vi "NI 5772 (AC) - Digitizer_vDirectDataSend (FPGA) Averaging (Working).vi"() -> ()   [LabVIEW 2020]
doc: "Example Description:\nThis example demonstrates how to enable Time Interleaved Sampling with the NI 5772 adapter module to achieve a sampling rate of 1.6GS/s. This example continuously acquires records of analog input data from the NI 5772 adapter module. It allows you to select an AI channel, trigger type, and record size. This VI must be compiled before it is run. \n\nRunning the VI:\nThis VI must be run from the NI 5772 - Getting Started (Host).vi. Refer to the host VI documentation for steps regarding running and configuring the FPGA VI. \n\nExecution Steps:\nRefer to the Block Diagram of this VI for execution comments."
uses:
  Controls/AI Trigger Type.ctl
  Controls/Aquire State.ctl
  <vilib>/Platform/TimedLoop/XDataNode/timing_clust.ctl
  <vilib>/Platform/TimedLoop/XDataNode/nitl_modes.ctl
  <vilib>/Platform/TimedLoop/XDataNode/wakeup.ctl
  Controls/DigitizerState.ctl
  <vilib>/rvi/Emulation/niFpgaGetClockAttributes.vi
  <vilib>/rvi/Emulation/niFpgaSctlEmulationGetInTimedLoop.vi
  <vilib>/rvi/Emulation/niFpgaEmulationReportErrorSimple.vi
  <vilib>/rvi/eio/common/nirviEmuTemplateMethod_errors.vi
  <vilib>/rvi/Emulation/niFpgaCriticalErrorInLSC.vi
  <vilib>/rvi/Emulation/niFpgaProcessEmulError.vi
  <vilib>/rvi/Emulation/niFpgaEmulationIsFPGAContextNoSignature.vi
  <vilib>/rvi/errors/niFpgaSetErrorForExecOnDevCompSimple.vi
  <vilib>/rvi/eio/common/nirviEmuReportErrorAndStop.vi
  <vilib>/rvi/DataTransferAndStorage/Container/Common/niFpgaContainerGetUniqueNameForEmu.vi
  <vilib>/rvi/FIFO/Fifo_Resource/nirvififoEmulationSetSize.vi
  <vilib>/rvi/FIFO/Fifo_Resource/nirviFifoEmulationQueueMgr.vi
  <instcachedir>/0/nirviFifoEmulationQueueMgr_E5CAEC123FF24DC58D834DCA3CDAA9B5.lvgen/nirviFifoEmulationQueueMgr_E5CAEC123FF24DC58D834DCA3CDAA9B5_004.vi
  <vilib>/Utility/error.llb/Clear Errors.vi
  <vilib>/rvi/FIFO/Fifo_Resource/nirvififoEmulationCreateLock.vi
  <vilib>/rvi/FIFO/Fifo_Resource/nirvififoEmulationObtainLock.vi
  <vilib>/rvi/FIFO/Fifo_Resource/nirvififoEmulationReleaseLock.vi
  <vilib>/rvi/occurrence/nirviWaitOnOccurrenceBase.vi
  <vilib>/rvi/errors/nirviReportUnexpectedCaseInternalError.vi
  <vilib>/rvi/errors/nirviReportUnexpectedCaseInternalError (U32).vi
  <instcachedir>/0/nirviFifoEmulationQueueMgr_E5CAEC123FF24DC58D834DCA3CDAA9B5.lvgen/nirviFifoEmulationQueueMgr_E5CAEC123FF24DC58D834DCA3CDAA9B5_000.vi
  <instcachedir>/0/nirviFifoEmulationQueueMgr_E5CAEC123FF24DC58D834DCA3CDAA9B5.lvgen/nirviFifoEmulationQueueMgr_E5CAEC123FF24DC58D834DCA3CDAA9B5_003.vi
  <vilib>/rvi/FIFO/Fifo_Resource/nirvififoEmulationDetermineInputValidOut.vi
  <vilib>/rvi/Memory/Memory_Emulation/nirvimemoryFastEmulation.vi
  <vilib>/rvi/Memory/Memory_Emulation/nirvimemoryEmulation.vi
  <vilib>/rvi/interface/RandomDataEmulation/niFpgaRandomDataHandleErrors.vi
  <instrlib>/_niInstr/Basic Elements/v1/FPGA/Private/Count Up U64.vi
  <vilib>/eio/EIONode/EIONode.xnode
  <vilib>/rvi/DataTransferAndStorage/Container/XNode/niFpgaContainer.xnode
  <vilib>/rvi/FIFO/Fifo_Resource/nirvififoEmulationRead.vi
  <vilib>/Platform/TimedLoop/XDataNode/XDataNode.xnode
  <vilib>/rvi/FIFO/Fifo_Resource/nirvififoEmulationWrite.vi
  <vilib>/rvi/interface/RandomDataEmulation/nirviRandomDataFpgaReadWriteTemplate.vi
  <vilib>/Platform/TimedLoop/XDataNode/XDNodeRunTimeDep.lvlib
  <instrlib>/_niInstr/Basic Elements/v1/FPGA/niInstr Basic Elements v1 FPGA.lvlib
panel:
  out "Read Size (Host)":u16=512 caption="Samples Per Trigger" min=1 step=1
  out "Trig Count":u64
  in  "Clear Count":bool
  in  "TrigIn Simulate":bool
  in  "vi/nGenTrig":bool
  in  "Arm Trigger":bool
  out "F to H FIFO Overflow?":bool caption="FIFO Overflow?"
  out "DataAlignmentFIFO":bool
  out "Aq to Trans FIFO Overflow?":bool caption="FIFO Overflow?"
  in  "Requested Samples Per Pixel":u16=512 caption="Samples Per Trigger" min=1 step=1
  in  "AvgCount_powerOf2":i16=1
  in  "Delay (us)":sgl
  in  "WaveSampleCount":sgl=256.0 format="%#_13g"
  in  "Wave Sampling Rate":sgl=200000000.0 format="%#_6p"
  in  "Trigger Level":i16
  in  "Trigger Type":T1
  out "AvgCount":u16=1
  out "Delay after Trig [cycles]":u16
  out "1/8th Samples Per Trigger":u16=512 caption="Samples Per Trigger" min=1 step=1
  out "WaitForWave\nCompletion [cycles]":u16
  in  "User Command Commit":bool
  in  "User Command":u8
  out "User Command Idle":bool
  out "User Command Status":u8
  in  "User Data 0":u16
  in  "User Data 1":u8
  out "PLL Locked":bool
  out "User Error":bool
  out "Configured?":bool
  # "Trigger Settings"
  # "FIFO Status"
  # "Analog Input"
  # "Clock Configuration"
  # "Resource Configuration"
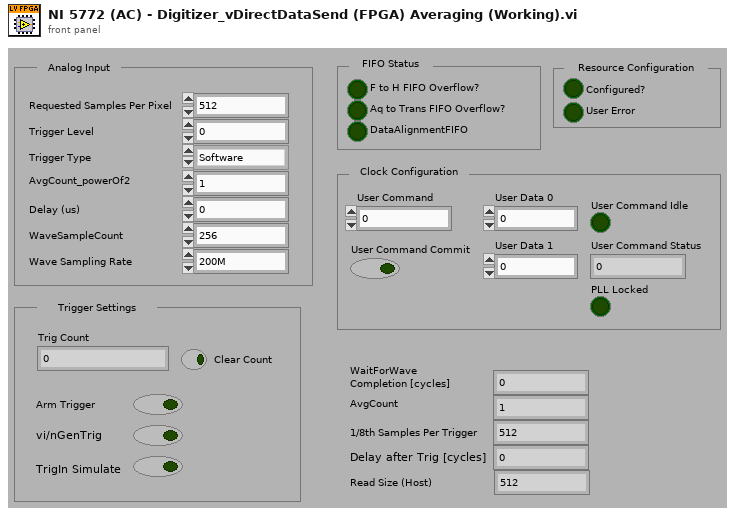
[diagram p1: front panel]
types:
  T1 = typedef "AI Trigger Type.ctl" = enum8{"Software", "Data Edge"}
  T2 = typedef "DigitizerState.ctl" = enum16{"Init", "Build/Clear Accumulator", "GetData", "SetData", "AverageCountCheck", "SendtoHost"}
  T3 = typedef "Aquire State.ctl" = enum8{"Idle", "Wait for Trigger", "AlignWave", "Hold Aquire", "Acquire", "WaitForWaveCompletion", "CheckAvg"}
  T4 = typedef "XDNodeRunTimeDep.lvlib/timing_clust.ctl" = cluster{"Expected End [f-1]":u64, "Actual End [f-1]":u64, "Finished Late? [f-1]":bool, "Expected End [i-1]":u64, "Actual End [i-1]":u64, "Finished Late? [i-1]":bool, "Expected Start [i]":u64, "Actual Start [i]":u64, "Expected Start [f]":u64, "Actual Start [f]":u64, "Source Name":string, "Structure Name":string, "Period":i64, "Deadline":i64, "Offset":i64, "Start":i64, "Priority":i32, "Timeout":i32, "Mode":T5, "Wakeup Reason":T6, "Error":errorcluster, "Source Type":string, "Secondary Source Type":string, "Global End Time":u64, "Global Start Time":u64, "Frame Duration":u64, "Iteration Duration":u64, "Assigned CPU":i32, "I/O Scan Engine Mode":u32}
  T5 = typedef "XDNodeRunTimeDep.lvlib/nitl_modes.ctl" = enum32{"No Change", "Process missed periods, maintain original phase", "Discard missed periods, maintain original phase", "Process missed periods, ignore original phase", "Discard missed periods, ignore original phase"}
  T6 = typedef "XDNodeRunTimeDep.lvlib/wakeup.ctl" = enum32{"Normal", "Aborted", "Asynchronous wakeup", "Timing source error", "Timed loop error", "Timeout"}
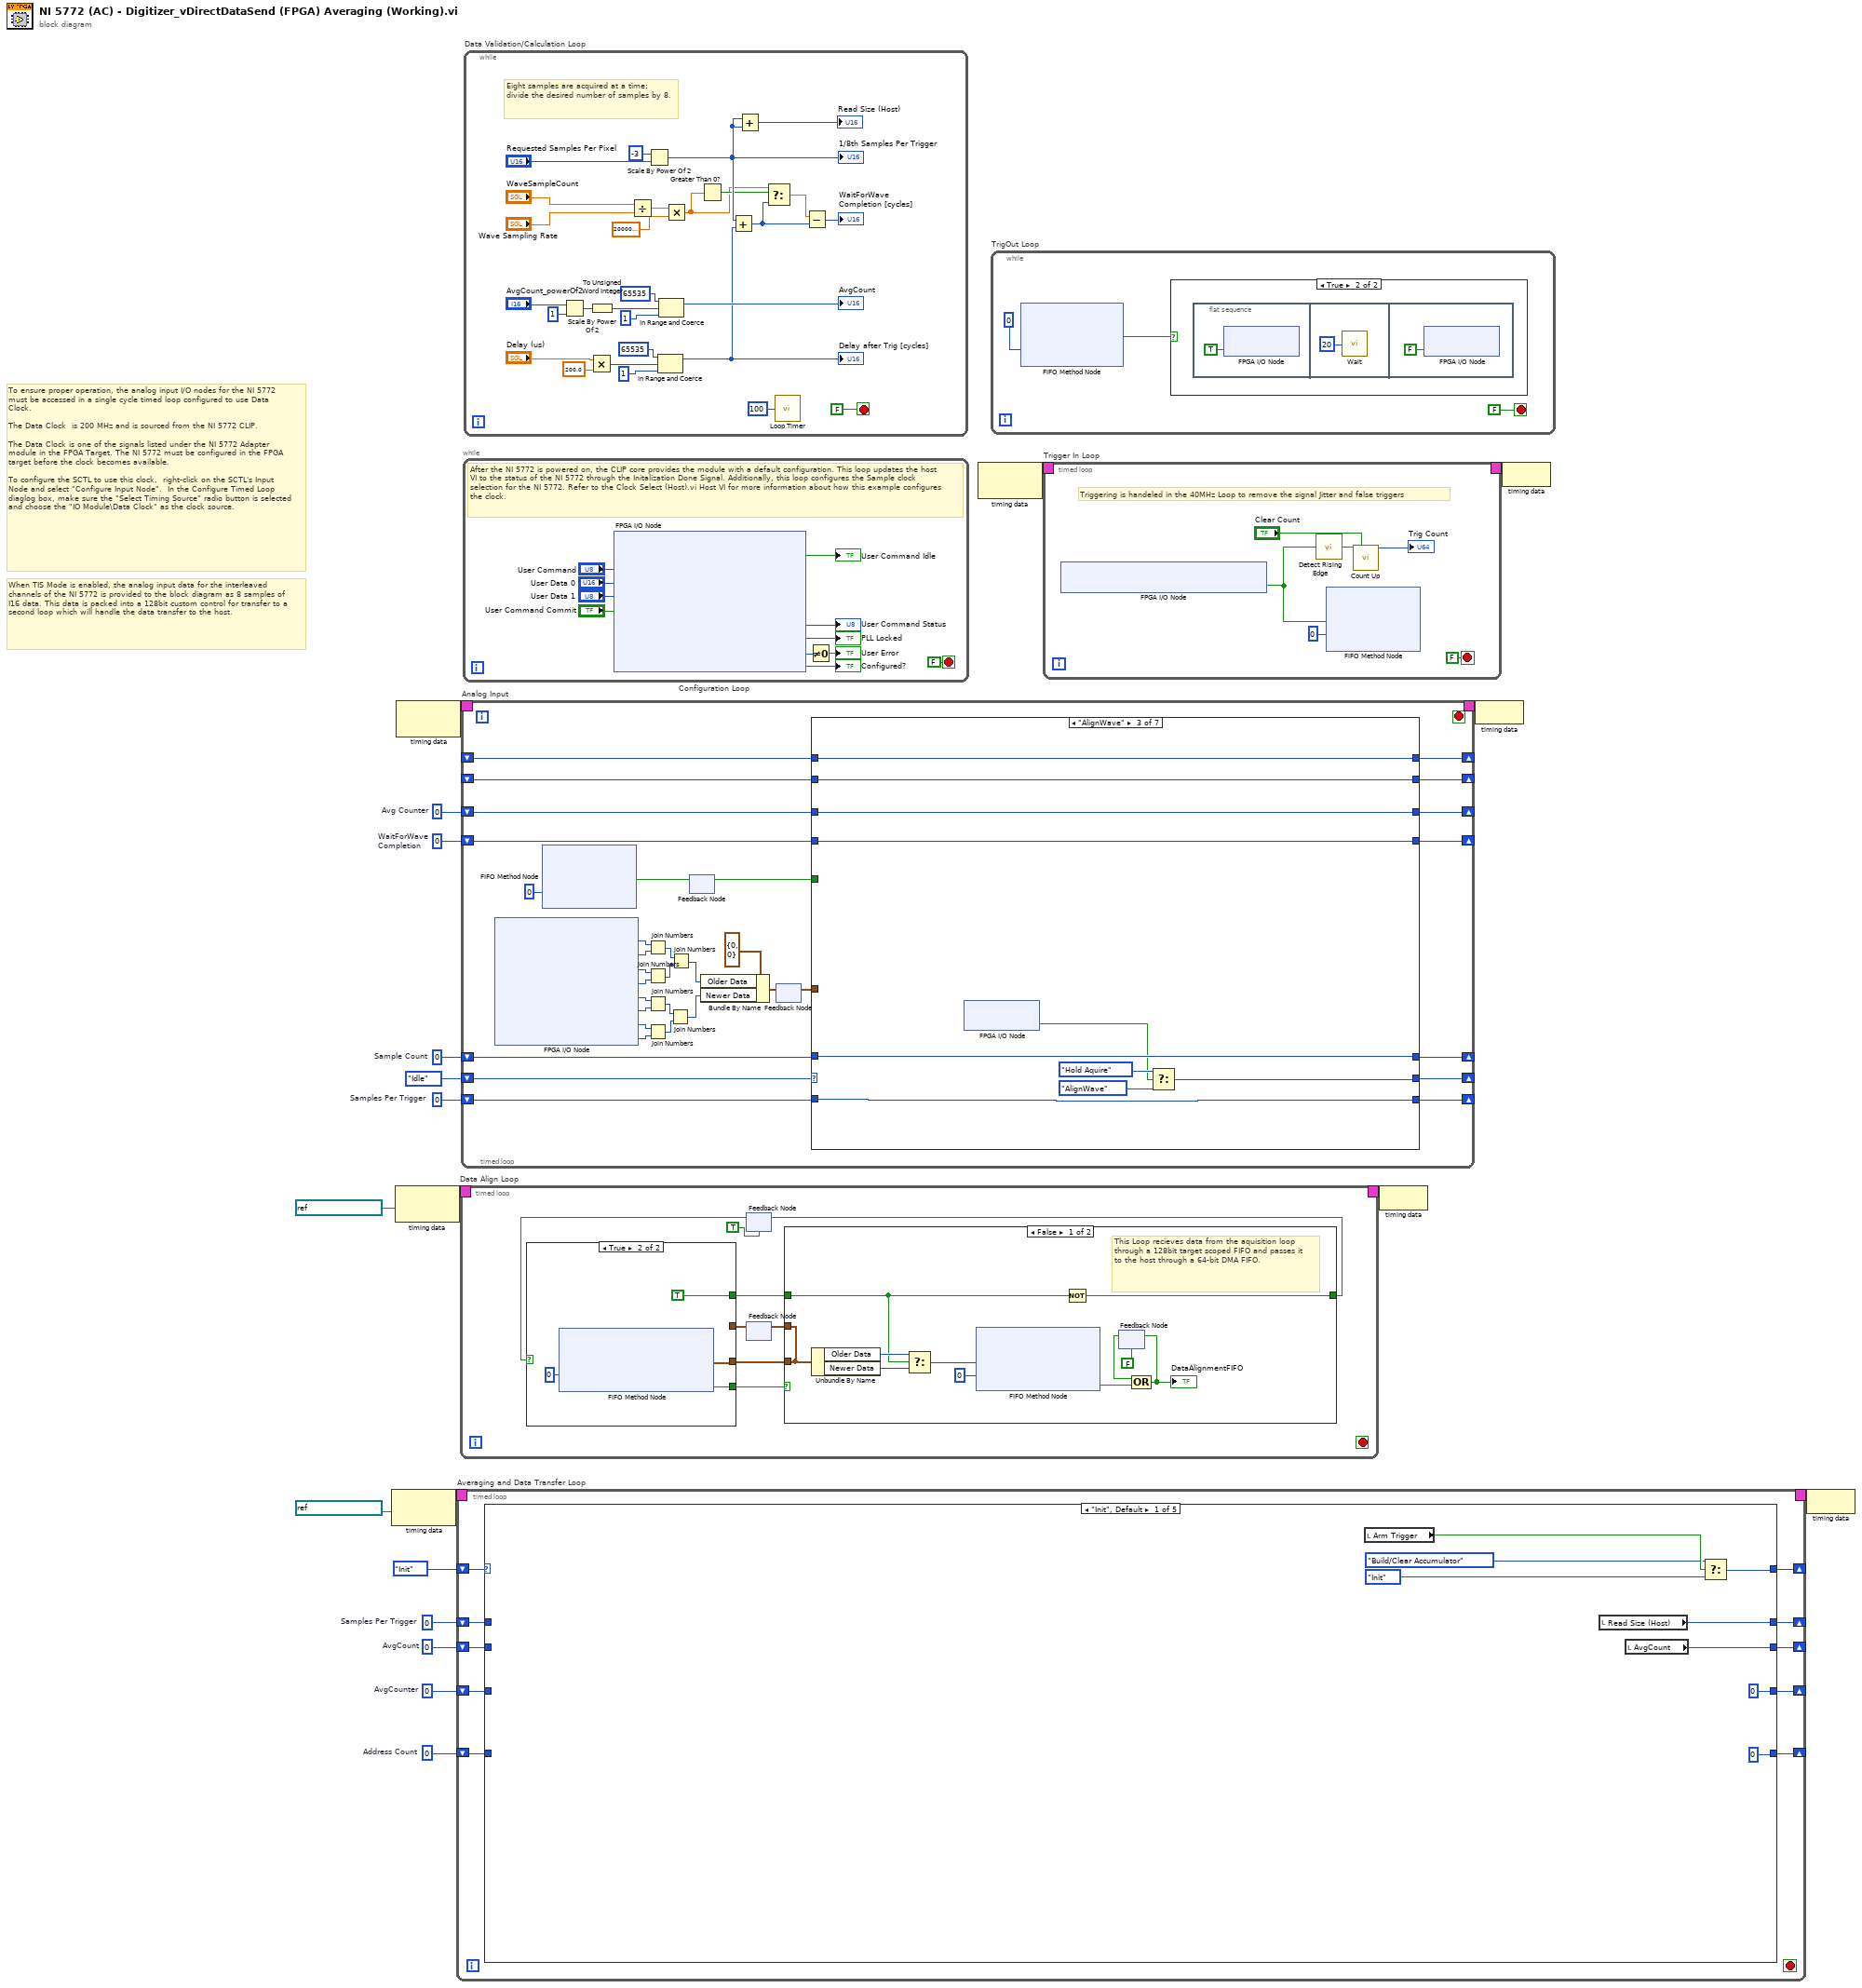
[diagram p0: block diagram]
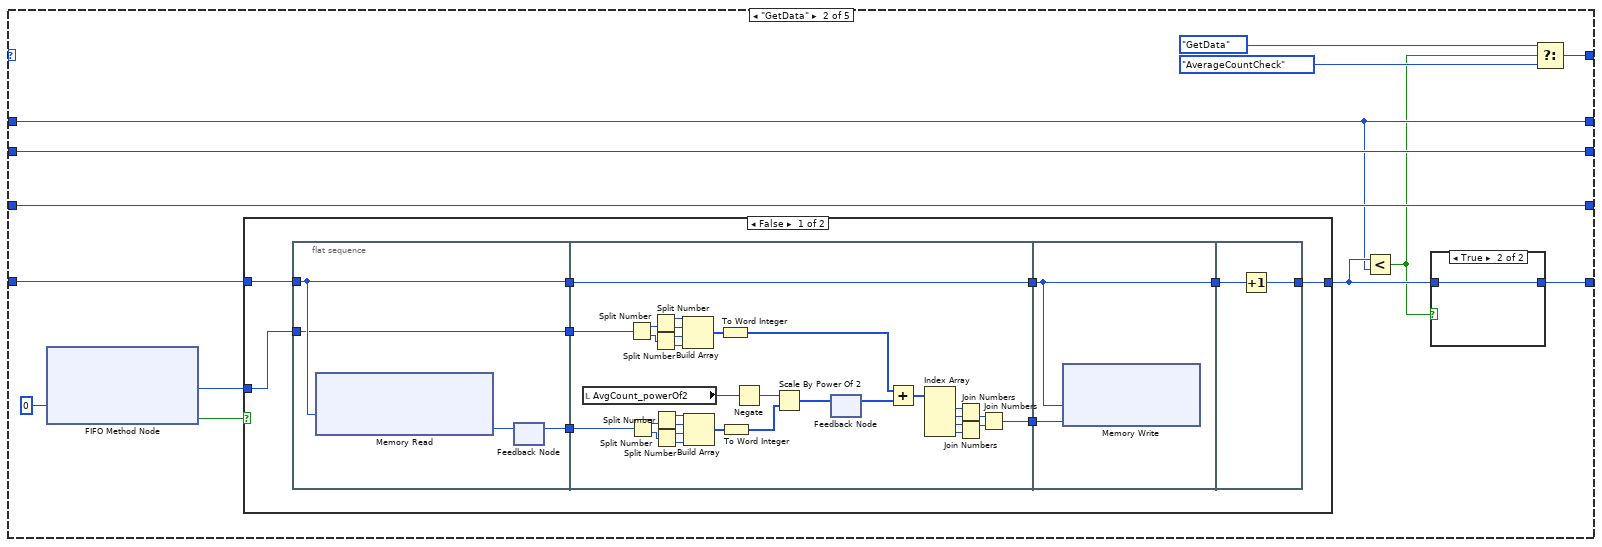
[diagram p2: hidden frame]
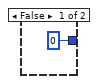
[diagram p3: hidden frame]
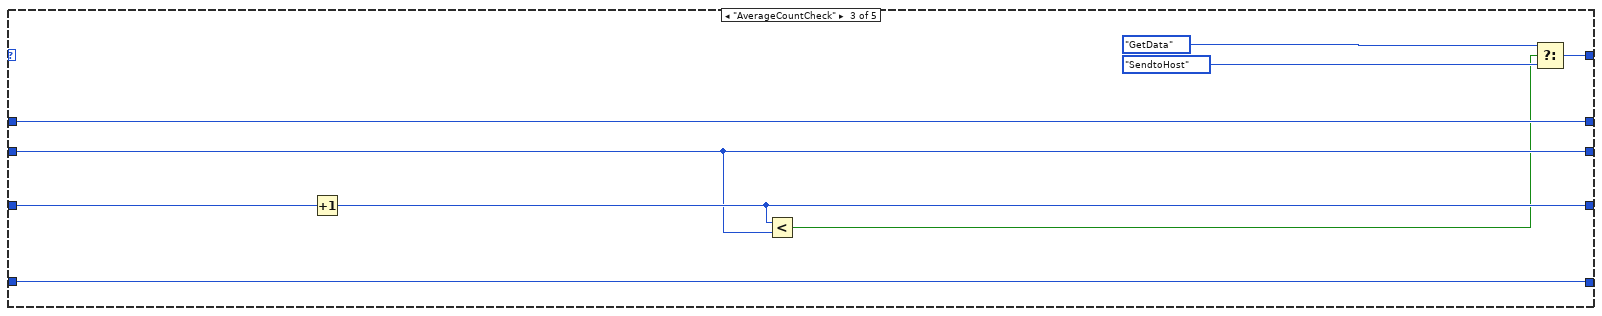
[diagram p5: hidden frame]
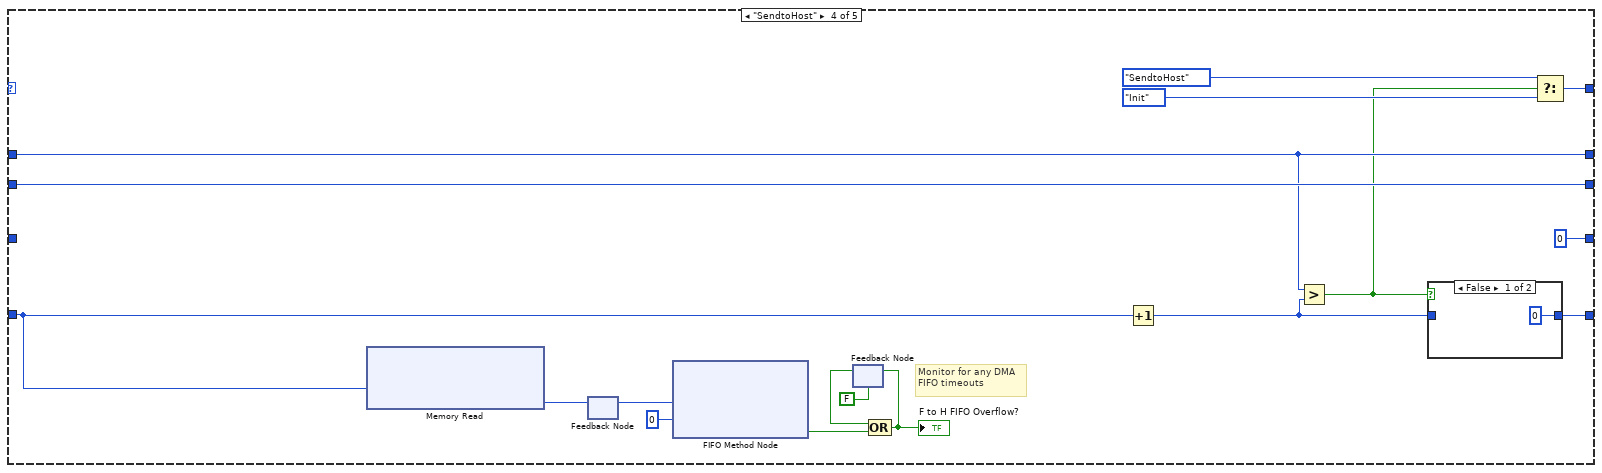
[diagram p6: hidden frame]
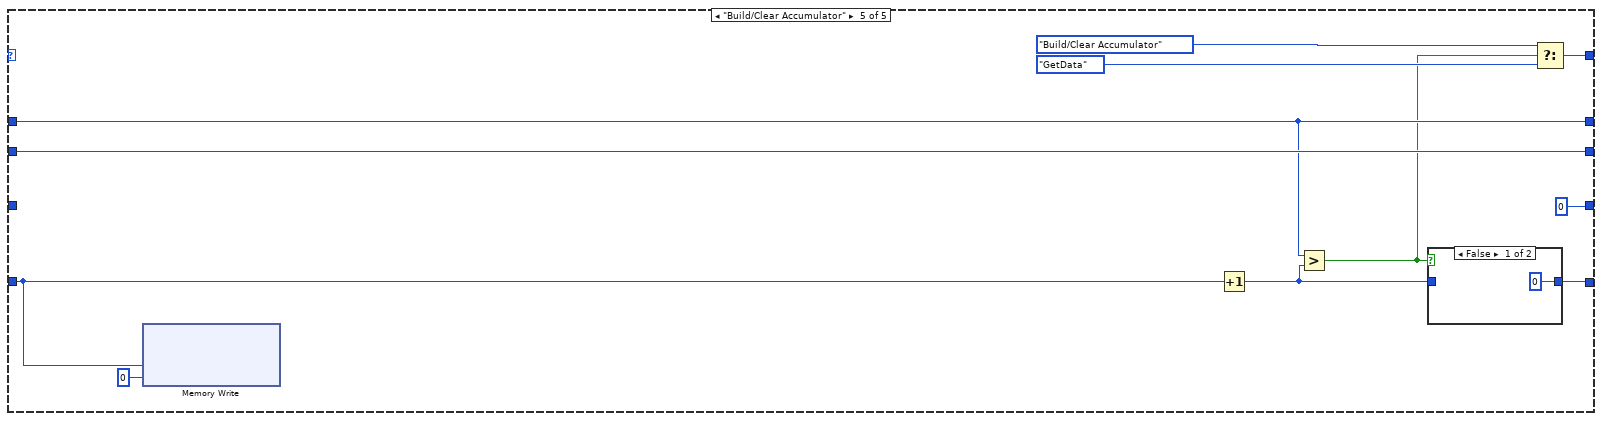
[diagram p8: hidden frame]
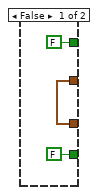
[diagram p10: hidden frame]
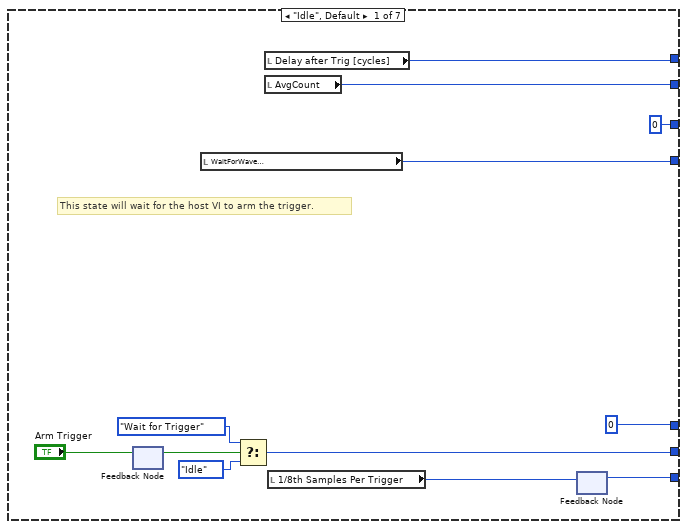
[diagram p13: hidden frame]
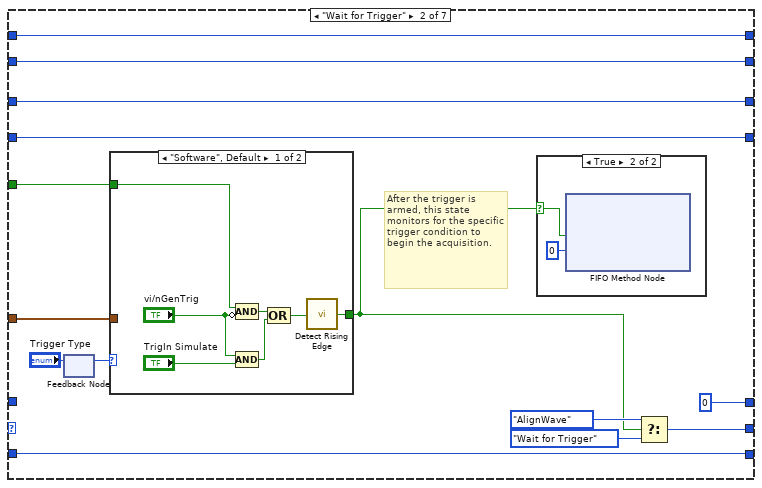
[diagram p14: hidden frame]
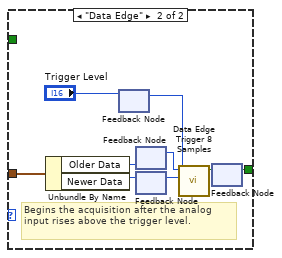
[diagram p16: hidden frame]
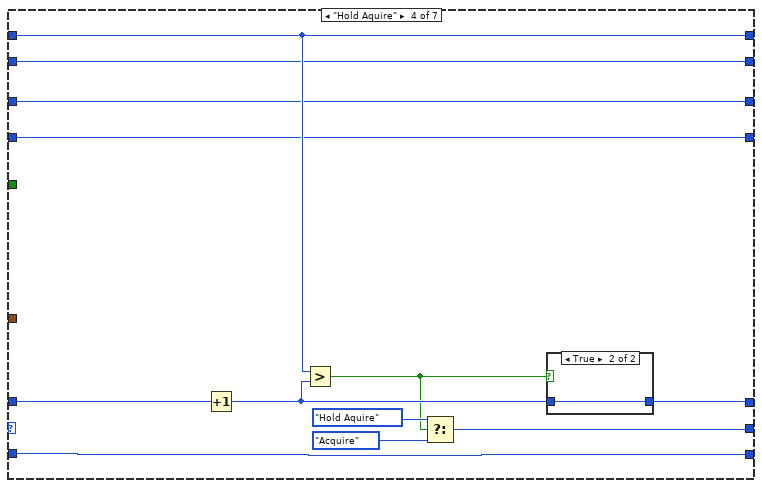
[diagram p17: hidden frame]
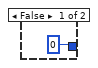
[diagram p18: hidden frame]
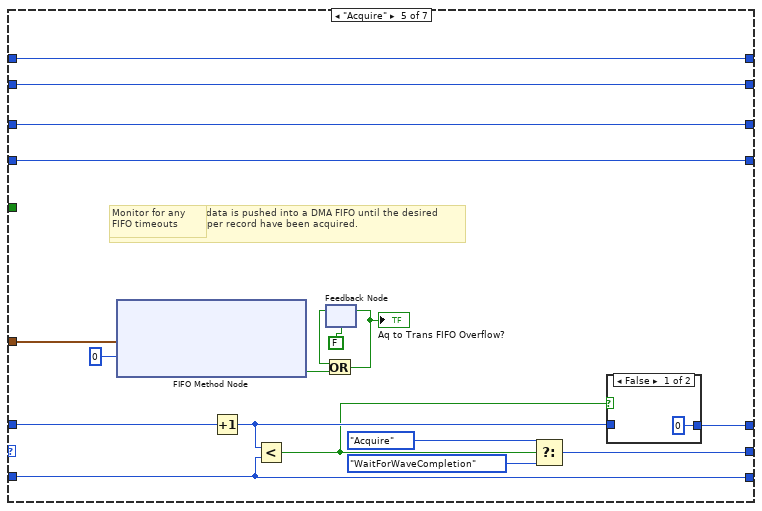
[diagram p19: hidden frame]
diagram:
  w6 = u16 0  # AvgCounter
  w5 = u32 0  # Address Count
  w4 = u16 0  # AvgCount
  w3 = u16 0  # Samples Per Trigger
  w12 = u16 0  # WaitForWave Completion
  w13 = u16 0  # Avg Counter
  w14 = u16 0  # Samples Per Trigger
  w15 = u16 0  # Sample Count
  # "When TIS Mode is enabled, the analog input data for the interleaved channels of the NI 5772 is provided to the block diagram as 8 samples of I16 data. This data is packed into a 128bit custom control for transfer to a second loop which will handle the data transfer to the host."
  # "To ensure proper operation, the analog input I/O nodes for the NI 5772 must be accessed in a single cycle timed loop configured to use Data Clock. \n\nThe Data Clock  is 200 MHz and is sourced from the NI 5772 CLIP.\n\nThe Data Clock is one of the signals listed under the NI 5772 Adapter module in the FPGA Target. The NI 5772 must be configured in the FPGA target before the clock becomes available. \n\nTo configure the SCTL to use this clock,  right-click on the SCTL's Input Node and select \"Configure Input Node\".  In the Configure Timed Loop diaglog box, make sure the \"Select Timing Source\" radio button is selected and choose the \"IO Module\\Data Clock\" as the clock source."
  n1 = node-c288(refnum<k21> "100 MHz Clock" ("Source Name")) -> (w8:T4)
  n2 = node-c288(refnum<k21> "100 MHz Clock" ("Source Name")) -> (w11:T4)
  n3 = node-c288() -> (w20:T4)  [unwired: 1 in]
  n4 = timed-loop "Averaging and Data Transfer Loop" {
    timing: w8 -> [_]
    timing-out: [_] -> w7
    shift-right: [w29] -> _
    shift-left: DigitizerState."Init" -> [w30]
    shift-right: [w28] -> _
    shift-left: w3 -> [w26]
    shift-right: [w27] -> _
    shift-left: w4 -> [w25]
    shift-right: [w23] -> _
    shift-left: w5 -> [w24]
    shift-right: [w21] -> _
    shift-left: w6 -> [w22]
    stop <- _ stop-if-true
    n5 = case shown="\"Init\", Default" w30 {
      tunnel: [w34 w49 w109 w125 w138] -> w29
      tunnel: [w32 w41 w107 w123 w136] -> w28
      tunnel: [w35 w48 w104 w128 w141] -> w27
      tunnel: w26 -> [_ w41 w107 w123 w136]
      tunnel: w25 -> [_ w48 w104 w128 w141]
      tunnel: w24 -> [_ w44 w108 w113 w132]
      tunnel: [u32 0 w43 w108 w124 w137] -> w23
      tunnel: [u16 0 w46 w105 u16 0 ("AvgCounter") u16 0 ("AvgCounter")] -> w21
      tunnel: w22 -> [_ w46 w106 _ _]
      frame "Init", Default {
        n6 = local read "Arm Trigger"() -> (w38:bool)
        n7 = local read "Read Size (Host)"() -> (w32:u16)
        n8 = local read "AvgCount"() -> (w35:u16)
        n9 = Select(t=DigitizerState."Build/Clear Accumulator", s=w38, f=DigitizerState."Init") -> (s? t:f=w34:T2)
      }
      frame "GetData" {
        n10 = xnode ("FIFO Method Node")("Timeout"=0) -> ("Element"=w45:u64, "Timed Out?"=w40:bool)  [unwired: 1 in, 1 out]
        n11 = case shown="False" w40 {
          tunnel: w45 -> [w59 _]
          tunnel: w44 -> [w61 w102]
          tunnel: [w58 w102] -> w42
          frame False {
            n12 = flat-sequence {
              tunnel: [w65] -> w62
              tunnel: w61 -> [w64]
              tunnel: w59 -> [w63]
              tunnel: [w64] -> w57
              tunnel: [w63] -> w55
              tunnel: w62 -> [w68]
              tunnel: [w87] -> w60
              tunnel: w57 -> [w86]
              tunnel: [w86] -> w56
              tunnel: w55 -> [w77]
              tunnel: w60 -> [w99]
              tunnel: w56 -> [w98]
              tunnel: [w98] -> w54
              tunnel: [w100] -> w58
              tunnel: w54 -> [w101]
              frame #0 {
                n13 = xnode ("Memory Read")("Address"=w64) -> ("Data"=w66:u64)  [unwired: 1 in, 1 out]
                n14 = feedback #1() -> (w65:u64)  [unwired: 1 in]
                n15 = feedback-in #1(w66) -> ()
              }
              frame #1 {
                n16 = local read "AvgCount_powerOf2"() -> (w96:i16)
                n17 = Split Number(x=w77) -> (hi(x)=w84:u32, lo(x)=w83:u32)
                n18 = Split Number(x=w68) -> (hi(x)=w69:u32, lo(x)=w70:u32)
                n19 = Split Number(x=w84) -> (hi(x)=w82:u16, lo(x)=w81:u16)
                n20 = Split Number(x=w83) -> (hi(x)=w80:u16, lo(x)=w79:u16)
                n21 = Split Number(x=w69) -> (hi(x)=w71:u16, lo(x)=w72:u16)
                n22 = Split Number(x=w70) -> (hi(x)=w73:u16, lo(x)=w74:u16)
                n23 = Build Array(w82, w81, w80, w79) -> (w78:u16[])
                n24 = Build Array(w71, w72, w73, w74) -> (w75:u16[])
                n25 = To Word Integer(number=w78) -> (16bit integer=w76:i16[])
                n26 = To Word Integer(number=w75) -> (16bit integer=w67:i16[])
                n27 = Negate(x=w96) -> (-x=w97:i16)
                n28 = Scale By Power Of 2(n=w97, x=w67) -> (x*2^n=w95:i16[])
                n29 = feedback-in #2(w95) -> ()
                n30 = feedback #2() -> (w85:i16[])  [unwired: 1 in]
                n31 = Add(x=w76, y=w85) -> (x+y=w88:i16[])
                n32 = Index Array(array=w88) -> (element #1=w91:i16, element #2=w92:i16, element #3=w93:i16, element #4=w94:i16)  [unwired: 4 in]
                n33 = Join Numbers(hi=w91, lo=w92) -> ((hi.lo)=w89:u32)
                n34 = Join Numbers(hi=w93, lo=w94) -> ((hi.lo)=w90:u32)
                n35 = Join Numbers(hi=w89, lo=w90) -> ((hi.lo)=w87:u64)
              }
              frame #2 {
                n36 = xnode ("Memory Write")("Address"=w98, "Data"=w99) -> ()  [unwired: 1 in, 1 out]
              }
              frame #3 {
                n37 = Increment(x=w101) -> (x+1=w100:u32)
              }
            }
          }
          frame True {
          }
        }
        n38 = Less?(x=w42, y=w41) -> (x < y?=w39:bool)
        n39 = case shown="True" w39 {
          tunnel: w42 -> [_ w53]
          tunnel: [u32 0 w53] -> w43
          frame False {
          }
          frame True {
          }
        }
        n40 = Select(t=DigitizerState."GetData", s=w39, f=DigitizerState."AverageCountCheck") -> (s? t:f=w49:T2)
      }
      frame "AverageCountCheck" {
        n41 = Increment(x=w106) -> (x+1=w105:u16)
        n42 = Less?(x=w105, y=w104) -> (x < y?=w103:bool)
        n43 = Select(t=DigitizerState."GetData", s=w103, f=DigitizerState."SendtoHost") -> (s? t:f=w109:T2)
      }
      frame "SendtoHost" {
        # "Monitor for any DMA FIFO timeouts"
        n44 = xnode ("Memory Read")("Address"=w113) -> ("Data"=w114:u64)  [unwired: 1 in, 1 out]
        n45 = feedback #3() -> (w112:u64)  [unwired: 1 in]
        n46 = feedback-in #3(w114) -> ()
        n47 = xnode ("FIFO Method Node")("Element"=w112, "Timeout"=0) -> ("Timed Out?"=w119:bool)  [unwired: 1 in, 1 out]
        n48 = feedback #4(FALSE) -> (w118:bool)
        n49 = Compound Arithmetic op=OR(w118, w119) -> (w120:bool)
        "F to H FIFO Overflow?" <- w120
        n50 = feedback-in #4(w120) -> ()
        n51 = Increment(x=w113) -> (x+1=w122:u32)
        n52 = Greater?(x=w123, y=w122) -> (0:w121:bool)
        n53 = case shown="False" w121 {
          tunnel: w122 -> [_ w130]
          tunnel: [u32 0 w130] -> w124
          frame False {
          }
          frame True {
          }
        }
        n54 = Select(t=DigitizerState."SendtoHost", s=w121, f=DigitizerState."Init") -> (s? t:f=w125:T2)
      }
      frame "Build/Clear Accumulator" {
        n55 = xnode ("Memory Write")("Address"=w132, "Data"=u64 0) -> ()  [unwired: 1 in, 1 out]
        n56 = Increment(x=w132) -> (x+1=w135:u32)
        n57 = Greater?(x=w136, y=w135) -> (0:w134:bool)
        n58 = case shown="False" w134 {
          tunnel: w135 -> [_ w143]
          tunnel: [u32 0 w143] -> w137
          frame False {
          }
          frame True {
          }
        }
        n59 = Select(t=DigitizerState."Build/Clear Accumulator", s=w134, f=DigitizerState."GetData") -> (s? t:f=w138:T2)
      }
    }
  }
  n60 = timed-loop "Data Align Loop" {
    timing: w11 -> [_]
    timing-out: [_] -> w10
    stop <- _ stop-if-true
    n61 = feedback #5(TRUE ("Timed Out?")) -> (w148:bool)
    n62 = feedback #6() -> (w149:cluster{"Older Data":u64, "Newer Data":u64})  [unwired: 1 in]
    n63 = case shown="True" w148 {
      tunnel: [w154 w157] -> w151
      tunnel: [FALSE ("Timed Out?") w158] -> w153
      tunnel: [FALSE ("Timed Out?") TRUE ("Timed Out?")] -> w152
      tunnel: w149 -> [w154 _]
      frame False {
      }
      frame True {
        n64 = xnode ("FIFO Method Node")("Timeout"=0) -> ("Element"=w157:cluster{"Older Data":u64, "Newer Data":u64}, "Timed Out?"=w158:bool)  [unwired: 1 in, 1 out]
      }
    }
    n65 = case shown="False" w153 {
      tunnel: [w169 w173] -> w147
      tunnel: w152 -> [w170 w173]
      tunnel: w151 -> [w168 w172]
      tunnel: [w168 w172] -> w150
      frame False {
        # "This Loop recieves data from the aquisition loop through a 128bit target scoped FIFO and passes it to the host through a 64-bit DMA FIFO."
        n66 = Unbundle By Name(w168) -> ("Older Data"=w171:u64, "Newer Data"=w167:u64)
        n67 = Select(t=w171, s=w170, f=w167) -> (s? t:f=w161:u64)
        n68 = xnode ("FIFO Method Node")("Element"=w161, "Timeout"=0) -> ("Timed Out?"=w163:bool)  [unwired: 1 in, 1 out]
        n69 = Not(x=w170) -> (.not. x?=w169:bool)
        n70 = feedback #7(FALSE) -> (w164:bool)
        n71 = Compound Arithmetic op=OR(w164, w163) -> (w162:bool)
        "DataAlignmentFIFO" <- w162
        n72 = feedback-in #7(w162) -> ()
      }
      frame True {
      }
    }
    n73 = feedback-in #5(w147) -> ()
    n74 = feedback-in #6(w150) -> ()
  }
  n75 = timed-loop "Analog Input" {
    timing: w20 -> [_]
    timing-out: [_] -> w19
    shift-right: [w208] -> _
    shift-left: Aquire_State."Idle" ("Acquire State") -> [w198]
    shift-right: [w209] -> _
    shift-left: w15 -> [w199]
    shift-right: [w207] -> _
    shift-left: w14 -> [w197]
    shift-right: [w184] -> _
    shift-left: _ -> [w183]
    shift-right: [w182] -> _
    shift-left: _ -> [w181]
    shift-right: [w179] -> _
    shift-left: w13 -> [w180]
    shift-right: [w177] -> _
    shift-left: w12 -> [w176]
    stop <- _ stop-if-true
    n76 = xnode "FPGA I/O Node"() -> ("IO Module\\AI 1 Data N-3"=w190:i16, "IO Module\\AI 0 Data N-3"=w189:i16, "IO Module\\AI 1 Data N-2"=w188:i16, "IO Module\\AI 0 Data N-2"=w187:i16, "IO Module\\AI 1 Data N-1"=w191:i16, "IO Module\\AI 0 Data N-1"=w192:i16, "IO Module\\AI 1 Data N"=w193:i16, "IO Module\\AI 0 Data N"=w194:i16)  [unwired: 8 in, 8 out]
    n77 = xnode ("FIFO Method Node")("Timeout"=0) -> ("Element"=w185:bool)  [unwired: 1 in, 2 out]
    n78 = Join Numbers(hi=w190, lo=w189) -> ((hi.lo)=w202:u32)
    n79 = Join Numbers(hi=w188, lo=w187) -> ((hi.lo)=w204:u32)
    n80 = Join Numbers(hi=w191, lo=w192) -> ((hi.lo)=w203:u32)
    n81 = Join Numbers(hi=w193, lo=w194) -> ((hi.lo)=w205:u32)
    n82 = Join Numbers(hi=w203, lo=w205) -> ((hi.lo)=w195:u64)
    n83 = Join Numbers(hi=w202, lo=w204) -> ((hi.lo)=w196:u64)
    n84 = feedback-in #8(w185) -> ()
    n85 = feedback #8() -> (w178:bool)  [unwired: 1 in]
    n86 = Bundle By Name(cluster=cluster{"Older Data":u64, "Newer Data":u64} {"Older Data"=0, "Newer Data"=0} ("Element"), "Older Data"=w196, "Newer Data"=w195) -> (w200:cluster{"Older Data":u64, "Newer Data":u64})
    n87 = feedback #9() -> (w206:cluster{"Older Data":u64, "Newer Data":u64})  [unwired: 1 in]
    n88 = feedback-in #9(w200) -> ()
    n89 = case shown="\"AlignWave\"" w198 {
      tunnel: [u16 0 u16 0 w259 w271 w280 w302 u16 0] -> w209
      tunnel: w199 -> [_ _ w259 w270 w295 w304 _]
      tunnel: [w218 w230 w262 w274 w294 w307 w318] -> w208
      tunnel: [w215 w234 w260 w272 w291 w305 w316] -> w207
      tunnel: w197 -> [_ w234 w260 w272 w291 w305 w316]
      tunnel: w206 -> [_ w233 _ _ w290 _ _]
      tunnel: w178 -> [_ w228 _ _ _ _ _]
      tunnel: [w214 w226 w258 w269 w284 w303 w315] -> w184
      tunnel: w183 -> [_ w226 w258 w269 w284 w303 w315]
      tunnel: [w213 w225 w257 w267 w283 w300 w313] -> w182
      tunnel: w181 -> [_ w225 w257 w267 w283 w300 w313]
      tunnel: [u16 0 ("Avg Count") w224 w256 w266 w282 w299 w312] -> w179
      tunnel: w180 -> [_ w224 w256 w266 w282 w299 w314]
      tunnel: [w210 w222 w254 w264 w278 w298 w309] -> w177
      tunnel: w176 -> [_ w222 w254 w264 w278 w298 w309]
      frame "Idle", Default {
        # "This state will wait for the host VI to arm the trigger."
        n90 = feedback-in #10("Arm Trigger") -> ()
        n91 = feedback #10() -> (w216:bool)  [unwired: 1 in]
        n92 = local read "WaitForWave\nCompletion [cycles]"() -> (w210:u16)
        n93 = Select(t=Aquire_State."Wait for Trigger" ("Acquire State"), s=w216, f=Aquire_State."Idle" ("Acquire State")) -> (s? t:f=w218:T3)
        n94 = local read "Delay after Trig [cycles]"() -> (w214:u16)
        n95 = local read "AvgCount"() -> (w213:u16)
        n96 = local read "1/8th Samples Per Trigger"() -> (w211:u16)
        n97 = feedback-in #11(w211) -> ()
        n98 = feedback #11() -> (w215:u16)  [unwired: 1 in]
      }
      frame "Wait for Trigger" {
        # "After the trigger is armed, this state monitors for the specific trigger condition to begin the acquisition."
        n99 = feedback-in #12("Trigger Type") -> ()
        n100 = feedback #12() -> (w227:T1)  [unwired: 1 in]
        n101 = case shown="\"Software\", Default" w227 {
          tunnel: w233 -> [_ w253]
          tunnel: [w244 w245] -> w223
          tunnel: w228 -> [w239 _]
          frame "Software", Default {
            n102 = Compound Arithmetic op=AND(w239, invert "vi/nGenTrig") -> (w243:bool)
            n103 = Compound Arithmetic op=AND("vi/nGenTrig", "TrigIn Simulate") -> (w241:bool)
            n104 = Compound Arithmetic op=OR(w243, w241) -> (w238:bool)
            n105 = call <instrlib>:"Detect Rising Edge.vi"("signal"=w238) -> ("edge detected"=w244:bool)  [unwired: 14 in]
          }
          frame "Data Edge" {
            # "Begins the acquisition after the analog input rises above the trigger level."
            n106 = Unbundle By Name(w253) -> ("Older Data"=w251:u64, "Newer Data"=w249:u64)
            n107 = feedback-in #13("Trigger Level") -> ()
            n108 = feedback #13() -> (w247:i16)  [unwired: 1 in]
            n109 = feedback-in #14(w251) -> ()
            n110 = feedback #14() -> (w246:u64)  [unwired: 1 in]
            n111 = feedback-in #15(w249) -> ()
            n112 = feedback #15() -> (w248:u64)  [unwired: 1 in]
            n113 = call "Data Edge Trigger 8 Samples.vi"("Trigger Level"=w247, "Newer Data In"=w248, "Older Data In"=w246) -> ("Trigger"=w252:bool)  [unwired: 8 in]
            n114 = feedback-in #16(w252) -> ()
            n115 = feedback #16() -> (w245:bool)  [unwired: 1 in]
          }
        }
        n116 = case shown="True" w223 {
          selector: w223 -> [_ w237]
          frame False {
          }
          frame True {
            n117 = xnode ("FIFO Method Node")("Element"=w237, "Timeout"=0) -> ()  [unwired: 1 in, 2 out]
          }
        }
        n118 = Select(t=Aquire_State."AlignWave" ("Acquire State"), s=w223, f=Aquire_State."Wait for Trigger") -> (s? t:f=w230:T3)
      }
      frame "AlignWave" {
        n119 = xnode "FPGA I/O Node"() -> ("PXI_Trig0"=w255:bool)  [unwired: 1 in, 1 out]
        n120 = Select(t=Aquire_State."Hold Aquire" ("Acquire State"), s=w255, f=Aquire_State."AlignWave" ("Acquire State")) -> (s? t:f=w262:T3)
      }
      frame "Hold Aquire" {
        n121 = Increment(x=w270) -> (x+1=w268:u16)
        n122 = Greater?(x=w269, y=w268) -> (0:w265:bool)
        n123 = Select(t=Aquire_State."Hold Aquire" ("Acquire State"), s=w265, f=Aquire_State."Acquire" ("Acquire State")) -> (s? t:f=w274:T3)
        n124 = case shown="True" w265 {
          tunnel: [u16 0 w277] -> w271
          tunnel: w268 -> [_ w277]
          frame False {
          }
          frame True {
          }
        }
      }
      frame "Acquire" {
        # "Monitor for any  FIFO timeouts"
        # "While in this state, data is pushed into a DMA FIFO until the desired number of samples per record have been acquired."
        n125 = xnode ("FIFO Method Node")("Element"=w290, "Timeout"=0) -> ("Timed Out?"=w285:bool)  [unwired: 1 in, 1 out]
        n126 = Increment(x=w295) -> (x+1=w281:u16)
        n127 = Less?(x=w281, y=w291) -> (x < y?=w279:bool)
        n128 = feedback #17(FALSE) -> (w286:bool)
        n129 = Or(x=w286, y=w285) -> (x .or. y?=w287:bool)
        "Aq to Trans FIFO Overflow?" <- w287
        n130 = feedback-in #17(w287) -> ()
        n131 = Select(t=Aquire_State."Acquire" ("Acquire State"), s=w279, f=Aquire_State."WaitForWaveCompletion" ("Acquire State")) -> (s? t:f=w294:T3)
        n132 = case shown="False" w279 {
          tunnel: w281 -> [_ w297]
          tunnel: [u16 0 w297] -> w280
          frame False {
          }
          frame True {
          }
        }
      }
      frame "WaitForWaveCompletion" {
        n133 = Increment(x=w304) -> (x+1=w302:u16)
        n134 = Greater?(x=w298, y=w302) -> (0:w301:bool)
        n135 = Select(t=Aquire_State."WaitForWaveCompletion" ("Acquire State"), s=w301, f=Aquire_State."CheckAvg" ("Acquire State")) -> (s? t:f=w307:T3)
      }
      frame "CheckAvg" {
        n136 = Increment(x=w314) -> (x+1=w312:u16)
        n137 = Greater?(x=w313, y=w312) -> (0:w310:bool)
        n138 = Select(t=Aquire_State."AlignWave" ("Acquire State"), s=w310, f=Aquire_State."Idle") -> (s? t:f=w318:T3)
        n139 = xnode ("FIFO Method Node")("Element"=w310, "Timeout"=0) -> ()  [unwired: 1 in, 2 out]
      }
    }
  }
  n140 = while "Configuration Loop" {
    stop <- FALSE stop-if-true
    # "After the NI 5772 is powered on, the CLIP core provides the module with a default configuration. This loop updates the host VI to the status of the NI 5772 through the Initalization Done Signal. Additionally, this loop configures the Sample clock selection for the NI 5772. Refer to the Clock Select (Host).vi Host VI for more information about how this example configures the clock."
    n141 = xnode "FPGA I/O Node"("IO Module\\User Command"="User Command", "IO Module\\User Data 0"="User Data 0", "IO Module\\User Data 1"="User Data 1", "IO Module\\User Command Commit"="User Command Commit") -> ("IO Module\\User Command Idle"=→"User Command Idle":bool, "IO Module\\User Command Status"=→"User Command Status":u8, "IO Module\\PLL Locked"=→"PLL Locked":bool, "IO Module\\User Error"=w328:u8, "IO Module\\Initialization Done"=→"Configured?":bool)  [unwired: 9 in, 9 out]
    n142 = Not Equal To 0?(x=w328) -> (x != 0?=→"User Error":bool)
  }
  n143 = while "Data Validation/Calculation Loop" {
    stop <- FALSE stop-if-true
    # "Eight samples are acquired at a time; divide the desired number of samples by 8."
    n144 = Scale By Power Of 2(n="AvgCount_powerOf2", x=1 ("Timeout")) -> (x*2^n=w359:i32)
    n145 = To Unsigned Word Integer(number=w359) -> (unsigned 16bit integer=w356:u16)
    n146 = Multiply(x="Delay (us)", y=sgl 200.0) -> (x*y=w352:u16)
    n147 = Divide(x="WaveSampleCount", y="Wave Sampling Rate") -> (x/y=w344:sgl)
    n148 = Scale By Power Of 2(n=i16 -3, x="Requested Samples Per Pixel") -> (x*2^n=w338:u16)
    "1/8th Samples Per Trigger" <- w338
    n149 = In Range and Coerce(upper limit=u16 65535, x=w352, lower limit=u16 1) -> (coerced(x)=w345:u16)  [unwired: 1 out]
    "Delay after Trig [cycles]" <- w345
    n150 = In Range and Coerce(upper limit=u16 65535, x=w356, lower limit=u16 1) -> (coerced(x)=→"AvgCount":u16)  [unwired: 1 out]
    n151 = Multiply(x=w344, y=sgl 200000000.0) -> (x*y=w335:sgl)
    n152 = Greater Than 0?(x=w335) -> (x > 0?=w336:bool)
    n153 = Add(x=w338, y=w345) -> (x+y=w334:u16)
    n154 = Add(x=w338, y=w338) -> (x+y=→"Read Size (Host)":u16)
    n155 = Select(t=w335, s=w336, f=w334) -> (s? t:f=w337:sgl)
    n156 = call "Loop Timer"("Count(uSec)"=u32 100 ("Count(mSec)")) -> ()  [unwired: 1 out]
    n157 = Subtract(x=w337, y=w334) -> (x-y=→"WaitForWave\nCompletion [cycles]":u16)
  }
  n158 = node-c288() -> (w18:T4)  [unwired: 1 in]
  n159 = while "TrigOut Loop" {
    stop <- FALSE stop-if-true
    n160 = xnode ("FIFO Method Node")("Timeout"=0) -> ("Element"=w362:bool)  [unwired: 1 in, 2 out]
    n161 = case shown="True" w362 {
      frame False {
      }
      frame True {
        n162 = flat-sequence {
          frame #0 {
            n163 = xnode "FPGA I/O Node"("PXI_Trig1"=TRUE) -> ()  [unwired: 1 in, 1 out]
          }
          frame #1 {
            n164 = call "Wait"("Count(Ticks)"=u32 20 ("Count(uSec)")) -> ()  [unwired: 1 out]
          }
          frame #2 {
            n165 = xnode "FPGA I/O Node"("PXI_Trig1"=FALSE) -> ()  [unwired: 1 in, 1 out]
          }
        }
      }
    }
  }
  n166 = timed-loop "Trigger In Loop" {
    timing: w18 -> [_]
    timing-out: [_] -> w17
    stop <- FALSE stop-if-true
    # "Triggering is handeled in the 40MHz Loop to remove the signal Jitter and false triggers"
    n167 = xnode "FPGA I/O Node"() -> ("IO Module\\Asynchronous Trigger Input"=w373:bool)  [unwired: 1 in, 1 out]
    n168 = call <instrlib>:"Detect Rising Edge.vi"("signal"=w373) -> ("edge detected"=w370:bool)  [unwired: 14 in]
    n169 = xnode ("FIFO Method Node")("Element"=w373, "Timeout"=0) -> ()  [unwired: 1 in, 2 out]
    n170 = call-poly <instrlib>:"Count Up.vi"("increment"=w370, "reset"="Clear Count") -> ("count out"=→"Trig Count":u64)  [unwired: 13 in]
  }
  n171 = node-c288(w10) -> ()
  n172 = node-c288(w19) -> ()
  n173 = node-c288(w17) -> ()
  n174 = node-c288(w7) -> ()
